vi "Client Side.vi"() -> ()   [LabVIEW 2021]
uses:
  gblV.vi
panel:
  out "Chanel":i32
  out "Volume":dbl(slide) scale=0.0..100.0
  out "Status":string
  in  "Stop":bool
  out "Doors":T1
  out "Curtains":T2 {"Vertical Pointer Slide 4" scale=0.0..10.0; "Vertical Pointer Slide 2" scale=0.0..10.0; "Vertical Pointer Slide" scale=0.0..10.0; "Curtain" scale=0.0..10.0; "Horizontal Pointer Slide 5" scale=0.0..10.0; "Horizontal Pointer Slide 4" scale=0.0..10.0; "Horizontal Pointer Slide 3" scale=0.0..10.0; "Horizontal Pointer Slide 2" scale=0.0..10.0; "Horizontal Pointer Slide" scale=0.0..10.0}
  out "Lights":T3
  # "Master Bedroom"
  # "Living Room"
  # "Kitchen"
  # "Bedroom 2"
  # "Balcony"
  # "Bedroom 1"
  # "Balcony 2"
  # "Balcony 1"
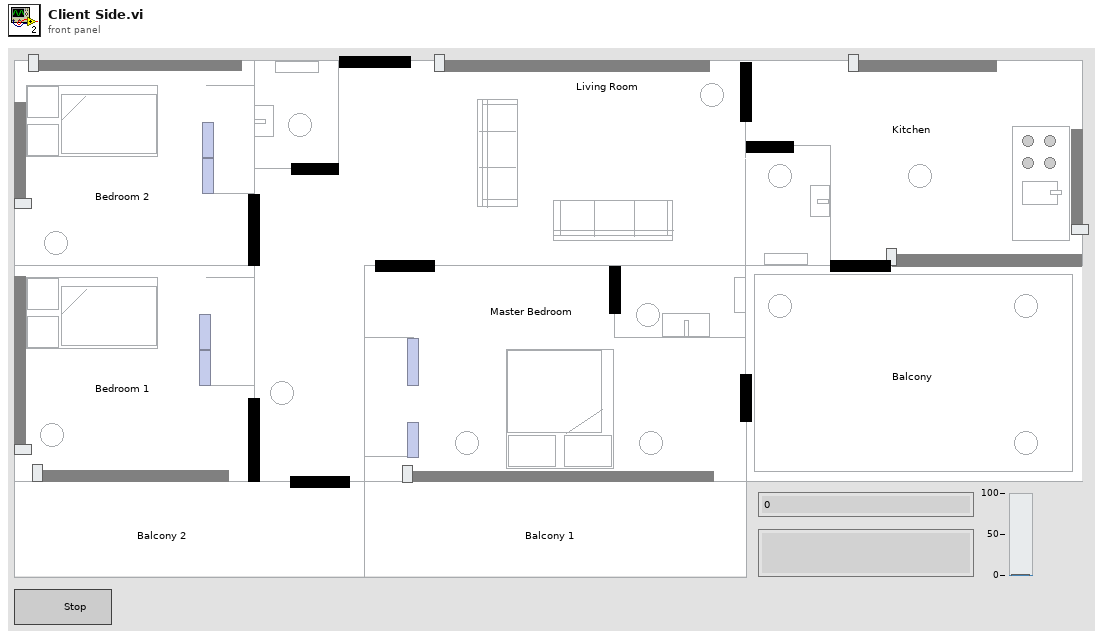
[diagram p1: front panel]
types:
  T1 = cluster{"Horizontal Slide Switch 3":bool, "Vertical Slide Switch 3":bool, "Vertical Slide Switch 5":bool, "Vertical Slide Switch 2":bool, "Vertical Slide Switch":bool, "Horizontal Slide Switch 4":bool, "Door":bool, "Horizontal Slide Switch 5":bool, "Horizontal Slide Switch 2":bool, "Vertical Slide Switch 4":bool, "Horizontal Slide Switch 6":bool, "Vertical Slide Switch 12":bool, "Vertical Slide Switch 14":bool, "Vertical Slide Switch 13":bool, "Vertical Slide Switch 6":bool, "Vertical Slide Switch 8":bool, "Vertical Slide Switch 7":bool, "Vertical Slide Switch 10":bool, "Vertical Slide Switch 9":bool, "Vertical Slide Switch 11":bool}
  T2 = cluster{"Horizontal Pointer Slide 3":dbl, "Horizontal Pointer Slide 2":dbl, "Vertical Pointer Slide 4":dbl, "Horizontal Pointer Slide":dbl, "Vertical Pointer Slide 2":dbl, "Curtain":dbl, "Horizontal Pointer Slide 5":dbl, "Vertical Pointer Slide":dbl, "Horizontal Pointer Slide 4":dbl}
  T3 = cluster{"Boolean 3":bool, "Boolean 4":bool, "Badroom 1":bool, "light":bool, "Boolean 9":bool, "Boolean 13":bool, "Boolean 8":bool, "Boolean 10":bool, "Boolean 11":bool, "Boolean 12":bool, "Boolean 5":bool, "Boolean 6":bool, "Boolean 7":bool}
  T4 = cluster{"Seek Back Button":bool, "Seek Forward Button":bool, "Remove Button":bool, "Add Button":bool, "Stop Button":bool, "Volume":dbl}
  T5 = cluster{"Curtains":cluster{"Horizontal Pointer Slide 3":dbl, "Horizontal Pointer Slide 2":dbl, "Vertical Pointer Slide 4":dbl, "Horizontal Pointer Slide":dbl, "Vertical Pointer Slide 2":dbl, "Curtain":dbl, "Horizontal Pointer Slide 5":dbl, "Vertical Pointer Slide":dbl, "Horizontal Pointer Slide 4":dbl}, "Lights":cluster{"Boolean 3":bool, "Boolean 4":bool, "Badroom 1":bool, "light":bool, "Boolean 9":bool, "Boolean 13":bool, "Boolean 8":bool, "Boolean 10":bool, "Boolean 11":bool, "Boolean 12":bool, "Boolean 5":bool, "Boolean 6":bool, "Boolean 7":bool}, "Doors":cluster{"Horizontal Slide Switch 3":bool, "Vertical Slide Switch 3":bool, "Vertical Slide Switch 5":bool, "Vertical Slide Switch 2":bool, "Vertical Slide Switch":bool, "Horizontal Slide Switch 4":bool, "Door":bool, "Horizontal Slide Switch 5":bool, "Horizontal Slide Switch 2":bool, "Vertical Slide Switch 4":bool, "Horizontal Slide Switch 6":bool, "Vertical Slide Switch 12":bool, "Vertical Slide Switch 14":bool, "Vertical Slide Switch 13":bool, "Vertical Slide Switch 6":bool, "Vertical Slide Switch 8":bool, "Vertical Slide Switch 7":bool, "Vertical Slide Switch 10":bool, "Vertical Slide Switch 9":bool, "Vertical Slide Switch 11":bool}, "TV":cluster{"Seek Back Button":bool, "Seek Forward Button":bool, "Remove Button":bool, "Add Button":bool, "Stop Button":bool, "Volume":dbl}}
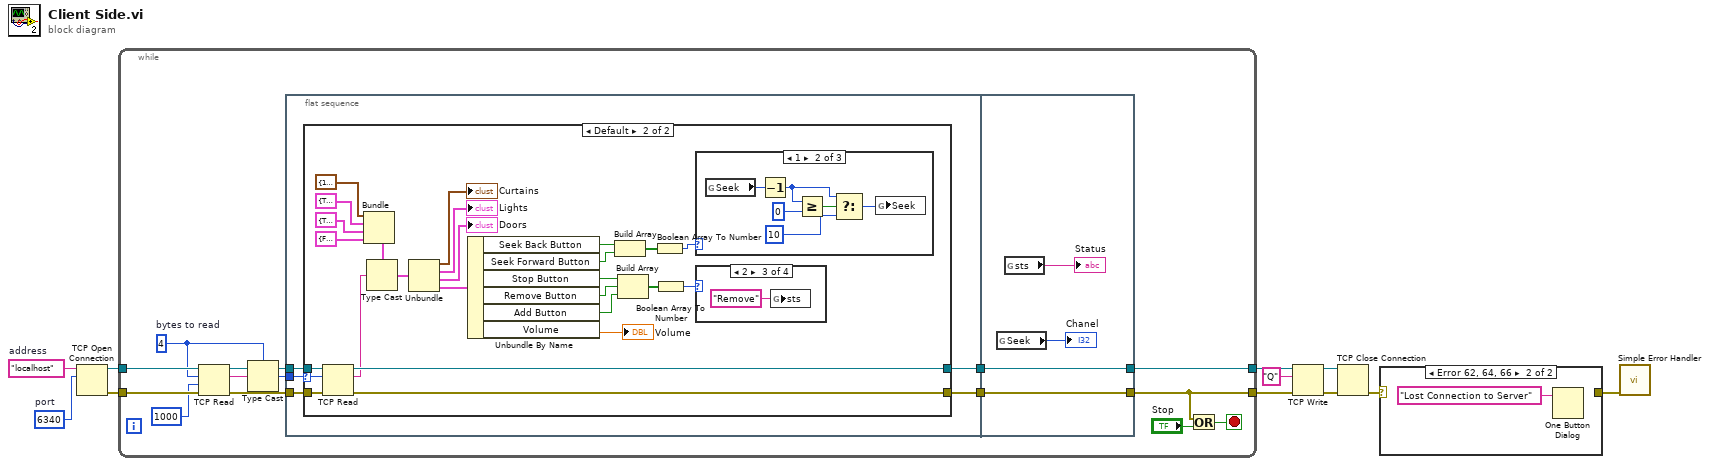
[diagram p0: block diagram]
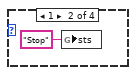
[diagram p5: hidden frame]
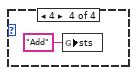
[diagram p6: hidden frame]
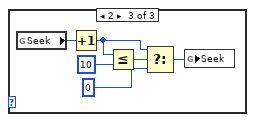
[diagram p8: hidden frame]
diagram:
  w1 = u16 6340  # port
  w2 = "localhost"  # address
  n1 = TCP Open Connection(address=w2, remote port or service name=w1) -> (connection ID=w11:refnum<k5>, error out=w10:errorcluster)  [unwired: 3 in]
  n2 = while {
    tunnel: w10 -> [w21]
    tunnel: w11 -> [w22]
    tunnel: [w18] -> w8
    tunnel: [w17] -> w6
    stop <- w19 stop-if-true
    w14 = 4  # bytes to read
    # "TCP Client Loop"
    n3 = TCP Read(connection ID=w22, bytes to read=w14, error in (no error)=w21, 9:1000 ("timeout ms (25000)")) -> (connection ID out=w24:refnum<k5>, data out=w25:string, error out=w23:errorcluster)  [unwired: 1 in]
    n4 = Type Cast(type=w14, x=w25) -> (*(type *) &x=w16:i32)
    n5 = flat-sequence {
      tunnel: w24 -> [w30]
      tunnel: w23 -> [w29]
      tunnel: w16 -> [w26]
      tunnel: [w28] -> w13
      tunnel: [w27] -> w12
      tunnel: [w76] -> w17
      tunnel: [w77] -> w18
      tunnel: w13 -> [w77]
      tunnel: w12 -> [w76]
      frame #0 {
        n6 = case shown="Default" w26 {
          selector: w26 -> [_ w53]
          tunnel: w30 -> [w32 w58]
          tunnel: w29 -> [w31 w57]
          tunnel: [w32 w56] -> w28
          tunnel: [w31 w55] -> w27
          frame ..0 {
            # "The server has not written any data"
          }
          frame Default {
            n7 = TCP Read(connection ID=w58, bytes to read=w53, error in (no error)=w57) -> (connection ID out=w56:refnum<k5>, data out=w54:string, error out=w55:errorcluster)  [unwired: 2 in]
            n8 = Bundle("Curtains"=T2 {"Horizontal Pointer Slide 3"=10.0, "Horizontal Pointer Slide 2"=10.0, "Vertical Pointer Slide 4"=10.0, "Horizontal Pointer Slide"=7.815533980582524, "Vertical Pointer Slide 2"=50.0, "Curtain"=10.0, "Horizontal Pointer Slide 5"=10.0, "Vertical Pointer Slide"=10.0, "Horizontal Pointer Slide 4"=34.0}, "Lights"=T3 {"Boolean 3"=TRUE, "Boolean 4"=TRUE, "Badroom 1"=TRUE, "light"=TRUE, "Boolean 9"=TRUE, "Boolean 13"=TRUE, "Boolean 8"=TRUE, "Boolean 10"=TRUE, "Boolean 11"=TRUE, "Boolean 12"=TRUE, "Boolean 5"=TRUE, "Boolean 6"=TRUE, "Boolean 7"=TRUE}, "Doors"=T1 {"Horizontal Slide Switch 3"=TRUE, "Vertical Slide Switch 3"=FALSE, "Vertical Slide Switch 5"=TRUE, "Vertical Slide Switch 2"=TRUE, "Vertical Slide Switch"=TRUE, "Horizontal Slide Switch 4"=TRUE, "Door"=TRUE, "Horizontal Slide Switch 5"=TRUE, "Horizontal Slide Switch 2"=TRUE, "Vertical Slide Switch 4"=TRUE, "Horizontal Slide Switch 6"=TRUE, "Vertical Slide Switch 12"=TRUE, "Vertical Slide Switch 14"=FALSE, "Vertical Slide Switch 13"=FALSE, "Vertical Slide Switch 6"=TRUE, "Vertical Slide Switch 8"=FALSE, "Vertical Slide Switch 7"=FALSE, "Vertical Slide Switch 10"=FALSE, "Vertical Slide Switch 9"=TRUE, "Vertical Slide Switch 11"=FALSE}, "TV"=T4 {"Seek Back Button"=FALSE, "Seek Forward Button"=FALSE, "Remove Button"=FALSE, "Add Button"=FALSE, "Stop Button"=FALSE, "Volume"=50.0}) -> (w49:T5)  [unwired: 1 in]
            n9 = Type Cast(type=w49, x=w54) -> (*(type *) &x=w48:T5)
            n10 = Unbundle(w48) -> ("Curtains"=→"Curtains":T2, "Lights"=→"Lights":T3, "Doors"=→"Doors":T1, "TV"=w42:T4)
            n11 = Unbundle By Name(w42) -> ("Seek Back Button"=w39:bool, "Seek Forward Button"=w44:bool, "Stop Button"=w36:bool, "Remove Button"=w35:bool, "Add Button"=w34:bool, "Volume"=→"Volume":dbl)
            n12 = Build Array(w39, w44) -> (w43:bool[])
            n13 = Build Array(w36, w35, w34) -> (w37:bool[])
            n14 = Boolean Array To Number(Boolean array=w43) -> (number=w38:u32)
            n15 = Boolean Array To Number(Boolean array=w37) -> (number=w33:u32)
            n16 = case shown="1" w38 {
              frame Default {
              }
              frame 1 {
                n17 = global read "gblV.vi" "Seek"() -> (w67:i32)
                n18 = Decrement(x=w67) -> (x-1=w64:i32)
                n19 = Greater Or Equal?(x=w64, y=0) -> (x >= y?=w65:bool)
                n20 = Select(t=w64, s=w65, f=10) -> (s? t:f=w62:i32)
                n21 = global write "gblV.vi" "Seek"(w62) -> ()
              }
              frame 2 {
                n22 = global read "gblV.vi" "Seek"() -> (w73:i32)
                n23 = Increment(x=w73) -> (x+1=w70:i32)
                n24 = Less Or Equal?(x=w70, y=10) -> (x <= y?=w71:bool)
                n25 = Select(t=w70, s=w71, f=0) -> (s? t:f=w68:i32)
                n26 = global write "gblV.vi" "Seek"(w68) -> ()
              }
            }
            n27 = case shown="2" w33 {
              frame Default {
              }
              frame 1 {
                n28 = global write "gblV.vi" "sts"("Stop" ("sts")) -> ()
              }
              frame 2 {
                n29 = global write "gblV.vi" "sts"("Remove" ("sts")) -> ()
              }
              frame 4 {
                n30 = global write "gblV.vi" "sts"("Add" ("sts")) -> ()
              }
            }
          }
        }
      }
      frame #1 {
        n31 = global read "gblV.vi" "Seek"() -> (→"Chanel":i32)
        n32 = global read "gblV.vi" "sts"() -> (→"Status":string)
      }
    }
    n33 = Or(x=w17, y="Stop") -> (x .or. y?=w19:bool)
  }
  n34 = TCP Write(connection ID=w8, data in="Q", error in (no error)=w6) -> (connection ID out=w9:refnum<k5>, error out=w7:errorcluster)  [unwired: 2 out]
  n35 = TCP Close Connection(connection ID=w9, error in (no error)=w7) -> (error out=w4:errorcluster)  [unwired: 1 in, 1 out]
  n36 = case shown="Error 62, 64, 66" w4 {
    selector: w4 -> [w78 _]
    tunnel: [w78 _] -> w3
    frame #0 {
    }
    frame #1 {
      n37 = One Button Dialog(message="Lost Connection to Server" ("Server Closed")) -> ()  [unwired: 1 in, 1 out]
    }
  }
  n38 = call <vilib>:"Simple Error Handler.vi"("error in (no error)"=w3) -> ()  [unwired: 4 in, 5 out]
